vi "My_Client.vi"() -> ()   [LabVIEW 2019]
uses:
  <vilib>/LabVIEW Open Source Project/MQTT Client/Client class/Client.lvclass/Client.ctl
  <vilib>/LabVIEW Open Source Project/MQTT Connection/MQTT_Base/Base Class/MQTT_Base.lvclass/MQTT_Base.ctl
  <vilib>/LabVIEW Open Source Project/MQTT TCP Connection/MQTT_TCP/Connection/TCPConnection.lvclass
  C:/Program Files (x86)/National Instruments/LabVIEW 2019/vi.lib/LabVIEW Open Source Project/MQTT Connection/MQTT_Connection/Connection/Connection.lvclass
  <vilib>/LabVIEW Open Source Project/MQTT Client/Client class/Client.lvclass
  C:/Program Files (x86)/National Instruments/LabVIEW 2019/vi.lib/LabVIEW Open Source Project/MQTT Connection/MQTT_Base/Base Class/MQTT_Base.lvclass
  <vilib>/LabVIEW Open Source Project/MQTT Control Packets/Control Packets/PUBLISH/PUBLISH.lvclass
  <vilib>/LabVIEW Open Source Project/MQTT Connection/MQTT_Base/Base Class/MQTT_Base.lvclass
panel:
  in  "Preiod":i32
  in  "Connection":bool
  in  "Stop Client":bool
  out "Published":bool
  out "Waveform Chart":dbl(graph)
  out "last error":errorcluster
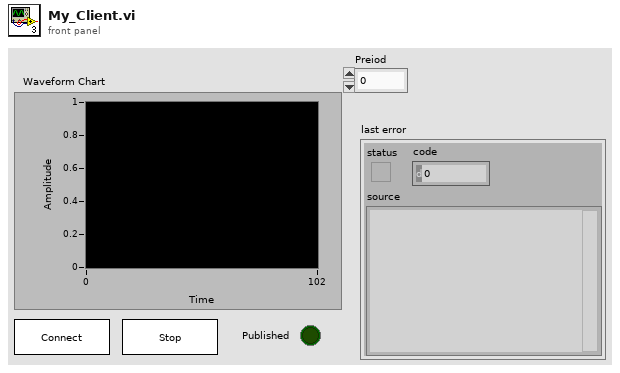
[diagram p1: front panel]
types:
  T1 = typedef "MQTT Client.lvlib/Client.lvclass/Public Events -- cluster.ctl" = cluster{"Connection Status":refnum<user-event>, "Connected":refnum<user-event>, "Application Message":refnum<user-event>}
  T2 = typedef "MQTT Base.lvlib/MQTT_Base.lvclass/Public Events -- cluster.ctl" = cluster{"Stop Event":refnum<user-event>, "Error Event":refnum<user-event>, "Inbound Message":refnum<user-event>}
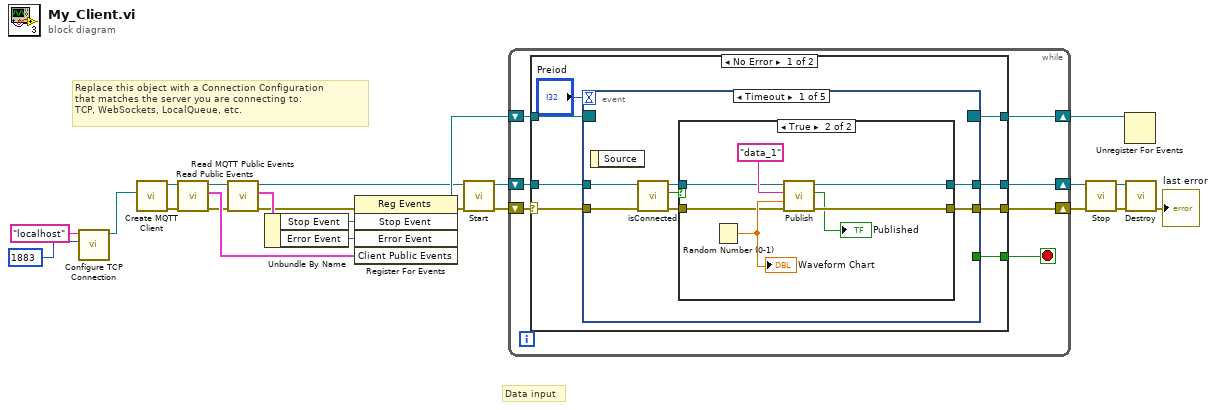
[diagram p0: block diagram]
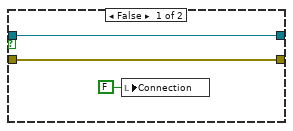
[diagram p2: hidden frame]
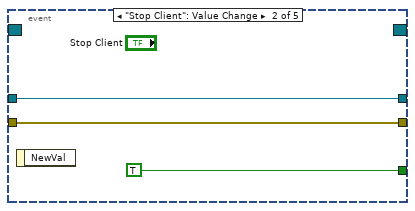
[diagram p3: hidden frame]
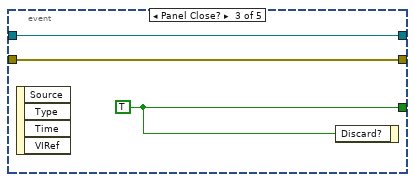
[diagram p4: hidden frame]
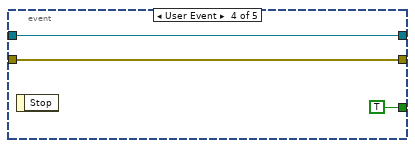
[diagram p5: hidden frame]
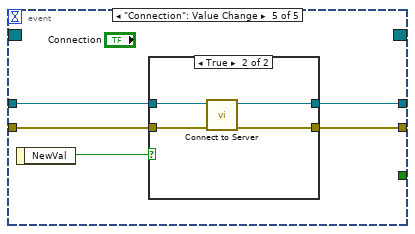
[diagram p6: hidden frame]
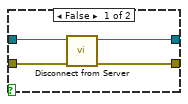
[diagram p7: hidden frame]
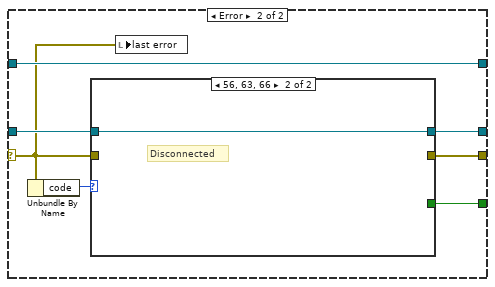
[diagram p8: hidden frame]
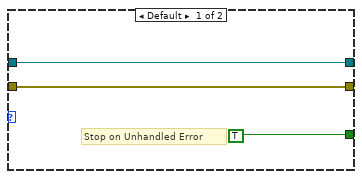
[diagram p9: hidden frame]
diagram:
  # "Data input"
  # "Replace this object with a Connection Configuration\nthat matches the server you are connecting to:\nTCP, WebSockets, LocalQueue, etc."
  n1 = call <vilib>:"Configure TCP Connection.vi"("remote port (80)"=u16 1883, "address (localhost)"="localhost") -> ("TCPConnection"=w3:refnum<class "TCPConnection.lvclass">)  [unwired: 8 in, 1 out]
  n2 = call <vilib>:"Create MQTT Client.vi"("Connection Configuration"=w3) -> ("error out"=w6:errorcluster, "Client out"=w4:refnum<class "Client.lvclass">)  [unwired: 9 in]
  n3 = call <vilib>:"Read Public Events.vi"("error in (no error)"=w6, "Client in"=w4) -> ("error out"=w7:errorcluster, "Client Public Events"=w9:T1, "Client out"=w5:refnum<class "Client.lvclass">)  [unwired: 7 in]
  n4 = call <vilib>:"Read MQTT Public Events.vi"("error in (no error)"=w7, "MQTT_Base in"=w5) -> ("error out"=w8:errorcluster, "MQTT Public Events"=w16:T2, "MQTT_Base out"=w11:refnum<class "Client.lvclass">)  [unwired: 7 in]
  n5 = Unbundle By Name(w16) -> ("Stop Event"=w14:refnum<user-event>, "Error Event"=w15:refnum<user-event>)
  n6 = register-events(error in=w8, w14, w15, w9) -> (reference out=w12:refnum<event-registration>, error out=w10:errorcluster)  [unwired: 1 in]
  n7 = call <vilib>:"Start.vi"("error in (no error)"=w10, "MQTT_Base in"=w11) -> ("error out"=w22:errorcluster, "MQTT_Base out"=w21:refnum<class "Client.lvclass">)  [unwired: 7 in, 1 out]
  n8 = while {
    shift-right: [w29] -> w13
    shift-left: w12 -> [w30]
    shift-right: [w26] -> w18
    shift-left: w21 -> [w27]
    shift-right: [w28] -> w20
    shift-left: w22 -> [w24]
    stop <- w25 stop-if-true
    n9 = case shown="No Error" w24 {
      selector: w24 -> [w32 w78]
      tunnel: w30 -> [w38 w84]
      tunnel: [w37 w84] -> w29
      tunnel: [w36 w80] -> w28
      tunnel: w27 -> [w35 w82]
      tunnel: [w34 w81] -> w26
      tunnel: [w33 w79] -> w25
      frame No Error {
        n10 = event shown="[0] Timeout" {
          selector: w38 -> [_ _ _ _ _]
          dyn-events: [_ _ _ _ _] -> w37
          timeout: "Preiod" -> [_ _ _ _ _]
          tunnel: w32 -> [w41 w57 w59 w64 w65]
          tunnel: [w44 w57 w59 w64 w66] -> w36
          tunnel: [_ TRUE w61 TRUE _] -> w33
          tunnel: w35 -> [w43 w58 w60 w62 w69]
          tunnel: [w45 w58 w60 w62 w67] -> w34
          event Timeout {
            n11 = event-data() -> ()  [unwired: 1 in, 1 out]
            n12 = call <vilib>:"isConnected.vi"("error in (no error)"=w41, "Client in"=w43) -> ("error out"=w40:errorcluster, "connected"=w39:bool, "Client out"=w42:refnum<class "Client.lvclass">)  [unwired: 7 in]
            n13 = case shown="True" w39 {
              tunnel: [w48 w54] -> w45
              tunnel: [w47 w53] -> w44
              tunnel: w42 -> [w48 w50]
              tunnel: w40 -> [w47 w49]
              frame False {
                n14 = local write "Connection"(FALSE ("Connection")) -> ()
              }
              frame True {
                n15 = Random Number (0-1)() -> (number: 0 to 1=w51:dbl)
                "Waveform Chart" <- w51
                n16 = call <vilib>:"Publish.vi"("error in (no error)"=w49, "Payload"=w51, "Topic Name (empty: Payload name)"="data_1", "Client in"=w50) -> ("error out"=w53:errorcluster, "Published"=→"Published":bool, "Client out"=w54:refnum<class "Client.lvclass">)  [unwired: 5 in]
              }
            }
          }
          event "Stop Client": Value Change {
            n17 = event-data() -> ()  [unwired: 1 in, 1 out]
          }
          event Panel Close? {
            w61 = TRUE
            n18 = event-data() -> ()  [unwired: 1 in, 4 out]
            n19 = event-data("Discard?"=w61) -> ()  [unwired: 1 in, 1 out]
          }
          event User Event {
            n20 = event-data() -> ()  [unwired: 1 in, 1 out]
          }
          event "Connection": Value Change {
            n21 = event-data() -> ("NewVal"=w68:bool)  [unwired: 1 in]
            n22 = case shown="True" w68 {
              tunnel: w69 -> [w73 w77]
              tunnel: [w72 w74] -> w67
              tunnel: [w71 w75] -> w66
              tunnel: w65 -> [w70 w76]
              frame False {
                n23 = call <vilib>:"Disconnect from Server.vi"("error in (no error)"=w70, "Client in"=w73) -> ("error out"=w71:errorcluster, "Client out"=w72:refnum<class "Client.lvclass">)  [unwired: 7 in, 1 out]
              }
              frame True {
                n24 = call <vilib>:"Connect to Server.vi"("error in (no error)"=w76, "Client in"=w77) -> ("error out"=w75:errorcluster, "Client out"=w74:refnum<class "Client.lvclass">)  [unwired: 6 in, 2 out]
              }
            }
          }
        }
      }
      frame Error {
        n25 = Unbundle By Name(w78) -> ("code"=w83:i32)
        n26 = case shown="56, 63, 66" w83 {
          tunnel: w82 -> [w87 w88]
          tunnel: [w87 w88] -> w81
          tunnel: w78 -> [w86 _]
          tunnel: [w86 _] -> w80
          tunnel: [TRUE _] -> w79
          frame Default {
            # "Stop on Unhandled Error"
          }
          frame 56, 63, 66 {
            # "Disconnected"
          }
        }
        n27 = local write "last error"(w78) -> ()
      }
    }
  }
  n28 = call <vilib>:"Stop.vi"("error in (no error)"=w20, "MQTT_Base in"=w18) -> ("error out"=w19:errorcluster, "MQTT_Base out"=w17:refnum<class "Client.lvclass">)  [unwired: 7 in, 1 out]
  n29 = Unregister For Events(event registration refnum=w13) -> ()  [unwired: 1 in, 1 out]
  n30 = call <vilib>:"Destroy.vi"("error in (no error)"=w19, "MQTT_Base in"=w17) -> ("error out"=→"last error":errorcluster)  [unwired: 8 in, 1 out]
